vi "add_JointCommand.vi"(4 "Names":string[](array[string]), 5 "Angles":dbl[](array[numeric]), 6 "Mode":enum16{"Position", "Velocity", "Effort"}(ring), 7 "msg in":string) -> (3 "msg out":string)   [LabVIEW 2013]
uses:
  Primitives/subs/i32Scalar.vi
  Primitives/subs/float64Array.vi
  Primitives/subs/stringArray.vi
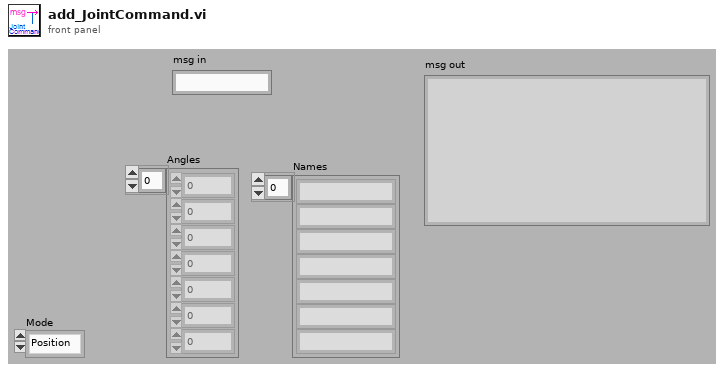
[diagram p1: front panel]
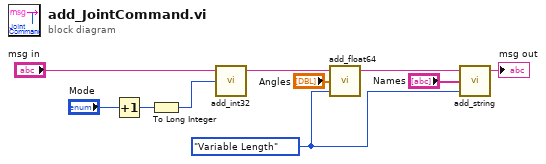
[diagram p0: block diagram]
diagram:
  w7 = enum16{"Fixed Length", "Variable Length"}."Variable Length" ("Array Type")
  n1 = Increment(x="Mode") -> (x+1=w4:enum16{"Position", "Velocity", "Effort"})
  n2 = To Long Integer(number=w4) -> (32bit integer=w1:i32)
  n3 = call-poly "add_int32.vi"("Numeric"=w1, "msg in"="msg in") -> ("msg out"=w2:string)  [unwired: 3 in]
  n4 = call-poly "add_float64.vi"("Array Type"=w7, "Array"="Angles", "msg in"=w2) -> ("msg out"=w9:string)  [unwired: 2 in]
  n5 = call-poly "add_string.vi"("Array Type"=w7, "Array"="Names", "msg in"=w9) -> ("msg out"=→"msg out":string)  [unwired: 2 in]
